vi "fronts_on.vi"(3 "in":bool) -> (0 "fall":bool, 1 "raise":bool)   [LabVIEW 2019, in "Logik.lvlib"]
uses:
  Logik.lvlib
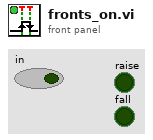
[diagram p1: front panel]
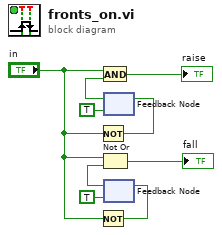
[diagram p0: block diagram]
diagram:
  n1 = Not(x="in") -> (.not. x?=w9:bool)
  n2 = Not(x="in") -> (.not. x?=w6:bool)
  n3 = feedback #1(TRUE) -> (w7:bool)
  n4 = And(x="in", y=w7) -> (x .and. y?=→"raise":bool)
  n5 = feedback-in #1(w9) -> ()
  n6 = feedback #2(TRUE) -> (w5:bool)
  n7 = Not Or(1:w5, 2:"in") -> (0:→"fall":bool)
  n8 = feedback-in #2(w6) -> ()
